vi "读取状态解析.vi"(8 "error in (no error)":errorcluster caption="错误输入（无错误）", 11 "Registers":u16[](array[numeric])) -> (0 "error out":errorcluster caption="错误输出", 3 "采样器状态":T1)   [LabVIEW 2016, in "超标留样集成.lvlib" / "德润DR803L超标留样.lvlib"]
panel:
  out "排空（瓶号）":u16
  out "停止采样泵":u16=1
  out "启动采样泵":u16=1
  # "0-4"
  # "8-14"
  # "48-52"
  # "60-64"
  # "54-59"
  # "5-7"
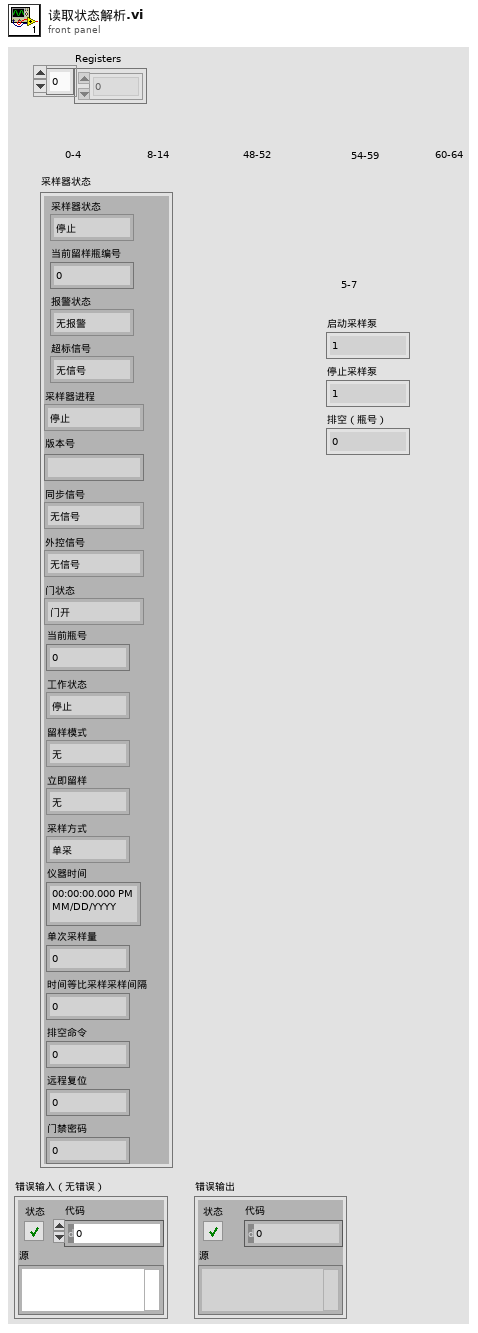
[diagram p1: front panel]
types:
  T1 = cluster{"采样器状态":enum16{"停止", "运行"}, "当前留样瓶编号":u16, "报警状态":enum16{"无报警", "留样失败报警"}, "超标信号":enum16{"无信号", "超标信号"}, "采样器进程":enum16{"停止", "待机", "定位校正", "移除瓶盖", "采样瓶排空", "管路润洗", "管存", "进样", "瓶盖密封", "管路排空", "调整采样位置", "采样结束", "采样瓶润洗", "瓶润洗排空"}, "版本号":string, "同步信号":enum16{"无信号", "同步信号"}, "外控信号":enum16{"无信号", "外控信号"}, "门状态":enum16{"门开", "门关"}, "当前瓶号":u16, "工作状态":enum16{"停止", "采样中"}, "留样模式":enum16{"无", "定时留样", "时间等比例", "超标留样", "同步留样", "外控留样"}, "立即留样":enum16{"无", "远程留样"}, "采样方式":enum16{"单采", "双重"}, "仪器时间":timestamp, "单次采样量":u16, "时间等比采样采样间隔":u16, "排空命令":u16, "远程复位":u16, "门禁密码":u16}
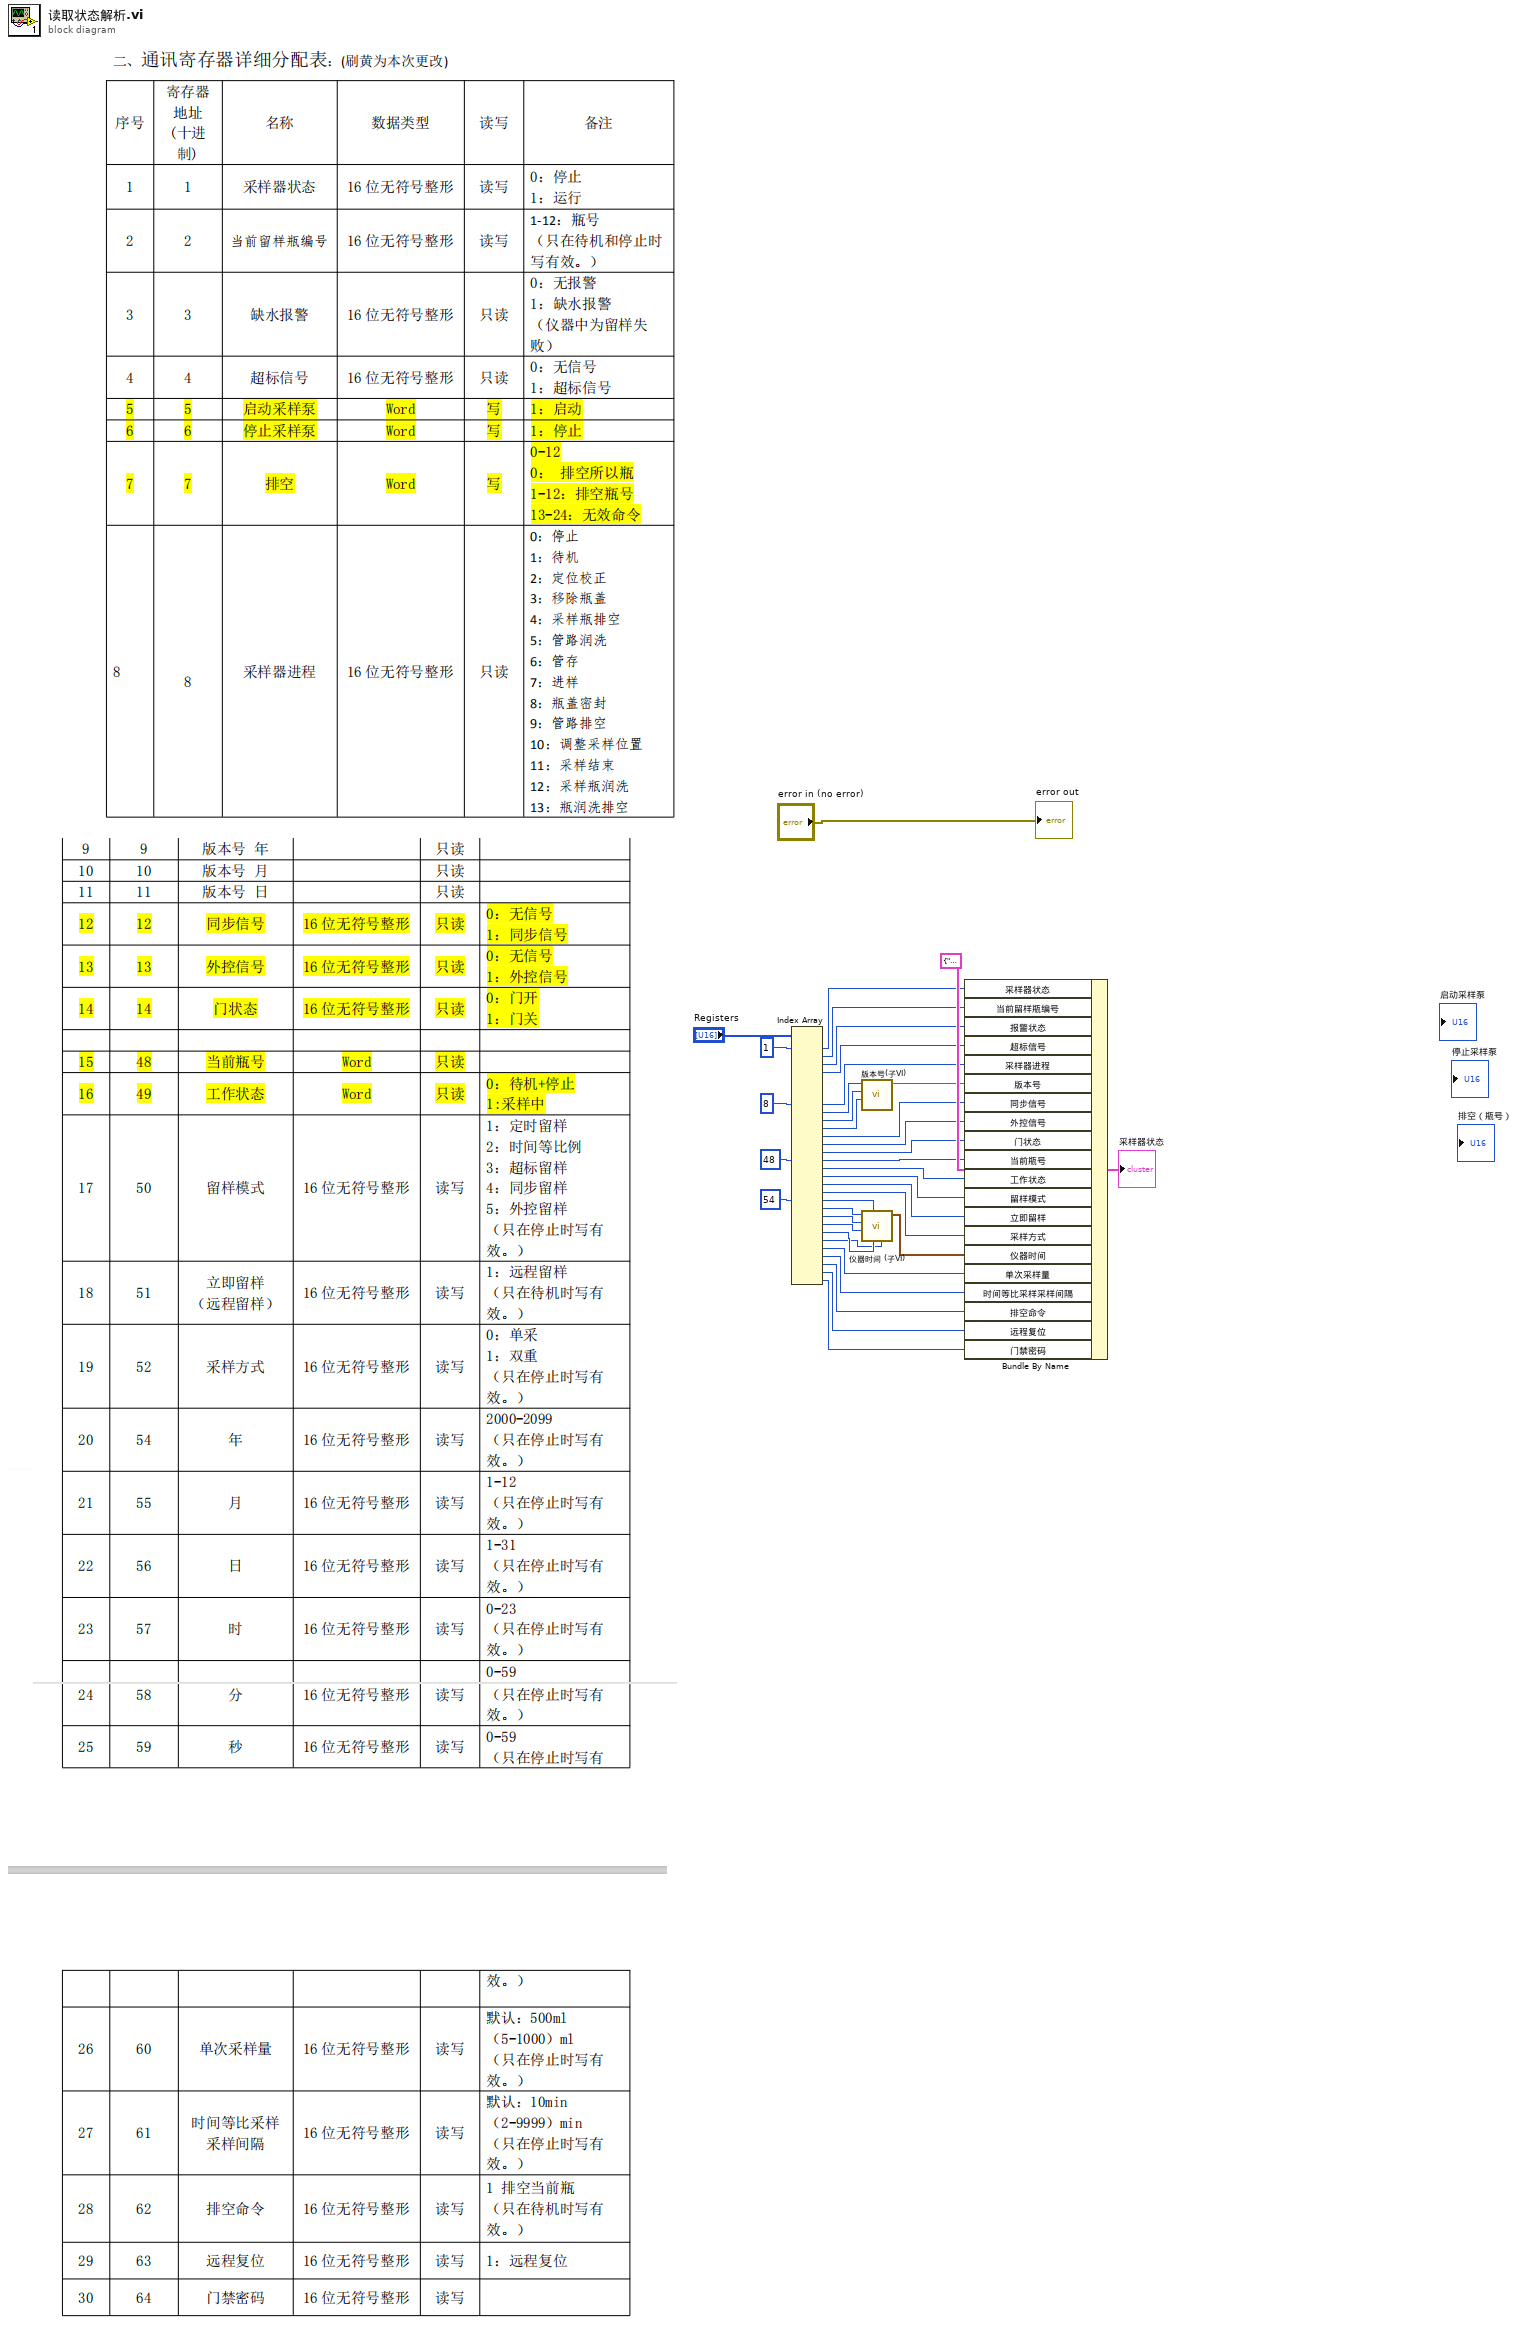
[diagram p0: block diagram]
diagram:
  n1 = Index Array(array="Registers", index #1=1 ("索引"), index #8=8 ("索引"), index #15=48 ("索引"), index #20=54 ("索引")) -> (element #1=w33:u16, element #2=w32:u16, element #3=w31:u16, element #4=w30:u16, element #8=w28:u16, element #9=w27:u16, element #10=w26:u16, element #11=w25:u16, element #12=w23:u16, element #13=w22:u16, element #14=w21:u16, element #15=w19:u16, element #16=w18:u16, element #17=w17:u16, element #18=w16:u16, element #19=w15:u16, element #20=w12:u16, element #21=w11:u16, element #22=w10:u16, element #23=w9:u16, element #24=w8:u16, element #25=w7:u16, element #26=w6:u16, element #27=w5:u16, element #28=w4:u16, element #29=w3:u16, element #30=w2:u16)  [unwired: 26 in, 3 out]
  n2 = call "版本号(子VI).vi"("数字 3"=w25, "数字 2"=w26, "数字"=w27) -> ("结果字符串"=w24:string)  [unwired: 8 in]
  n3 = call "仪器时间 (子VI).vi"("秒"=w7, "分"=w8, "年"=w12, "时"=w9, "日"=w10, "月"=w11) -> ("time stamp"=w13:timestamp)  [unwired: 5 in]
  n4 = Bundle By Name(cluster=T1 {"采样器状态"=enum."停止", "当前留样瓶编号"=0, "报警状态"=enum."留样失败报警", "超标信号"=enum."无信号", "采样器进程"=enum."采样瓶润洗", "版本号"="", "同步信号"=enum."无信号", "外控信号"=enum."无信号", "门状态"=enum."门关", "当前瓶号"=65535, "工作状态"=enum."采样中", "留样模式"=enum."定时留样", "立即留样"=enum."远程留样", "采样方式"=enum."单采", "仪器时间"=timestamp(0 s since 1904-01-01), "单次采样量"=65535, "时间等比采样采样间隔"=65535, "排空命令"=65535, "远程复位"=65535, "门禁密码"=65535} ("采样器状态"), "采样器状态"=w33, "当前留样瓶编号"=w32, "报警状态"=w31, "超标信号"=w30, "采样器进程"=w28, "版本号"=w24, "同步信号"=w23, "外控信号"=w22, "门状态"=w21, "当前瓶号"=w19, "工作状态"=w18, "留样模式"=w17, "立即留样"=w16, "采样方式"=w15, "仪器时间"=w13, "单次采样量"=w6, "时间等比采样采样间隔"=w5, "排空命令"=w4, "远程复位"=w3, "门禁密码"=w2) -> (→"采样器状态":T1)
  "error out" <- "error in (no error)"
